vi "mock.vi"() -> ()   [LabVIEW 2017]
uses:
  refnum_array_cluster.ctl
  Utility Sub VIs/pulse_generator_data_charts.ctl
  Utility Sub VIs/pulse_generator_data.ctl
  Utility Sub VIs/pressure_temp_mixture.ctl
  Utility Sub VIs/diode_charts.ctl
panel:
  out "Diode Charts":T1
  out "Pressure/Temperature/Mixture Properties":T2
  out "Measurements":T3={"PG Abs Pressure"=119484.80284900061, "Vapor Temperature"=19.805676371442082, "Liquid Temperature"=19.52526901660894, "Tinlet"=121.24568157832624, "Tsectwo"=119.96937909943745, "TS Abs Pressure W1"=121.24568157832624, "TS Abs Pressure W7"=119.96937909943745, "W1-4 dP[Pa]"=19.52526901660894, "W1-7 dP[Pa]"=119.96937909943745, "W1-7 dP[Pa] Fast"=119.96937909943745, "PG Venturi dP [Pa]"=119.96937909943745, "Vapor Line Pitot dP [Pa]"=119.96937909943745, "Tsecthree"=19.191961040039615, "Toutlet"=19.148186089917207, "TS Ext"=18.97439824494449, "Vapor Sat Pressure"=121.24568157832624, "Liquid Sat Pressure"=119.96937909943745, "PG Mass Flow Rate"=nan, "Vapor Line Mass Flow"=119.96937909943745}
  out "Pulse Generator Charts":T4
  # "Saturation\nPressure [Pa]"
  # "Saturation\nTemperature [C]"
  # "Pressure [Pa]"
  # "Temperature [C]"
  # "Liquid Tank"
  # "Separator"
  # "Liquid Inlet"
  # "Vapor Tank"
  # "Vapor Inlet"
  # "Test Section"
  # "Upper Dev Section"
  # "Lower Dev Section"
  # "Test Section"
  # "Pulse Gen"
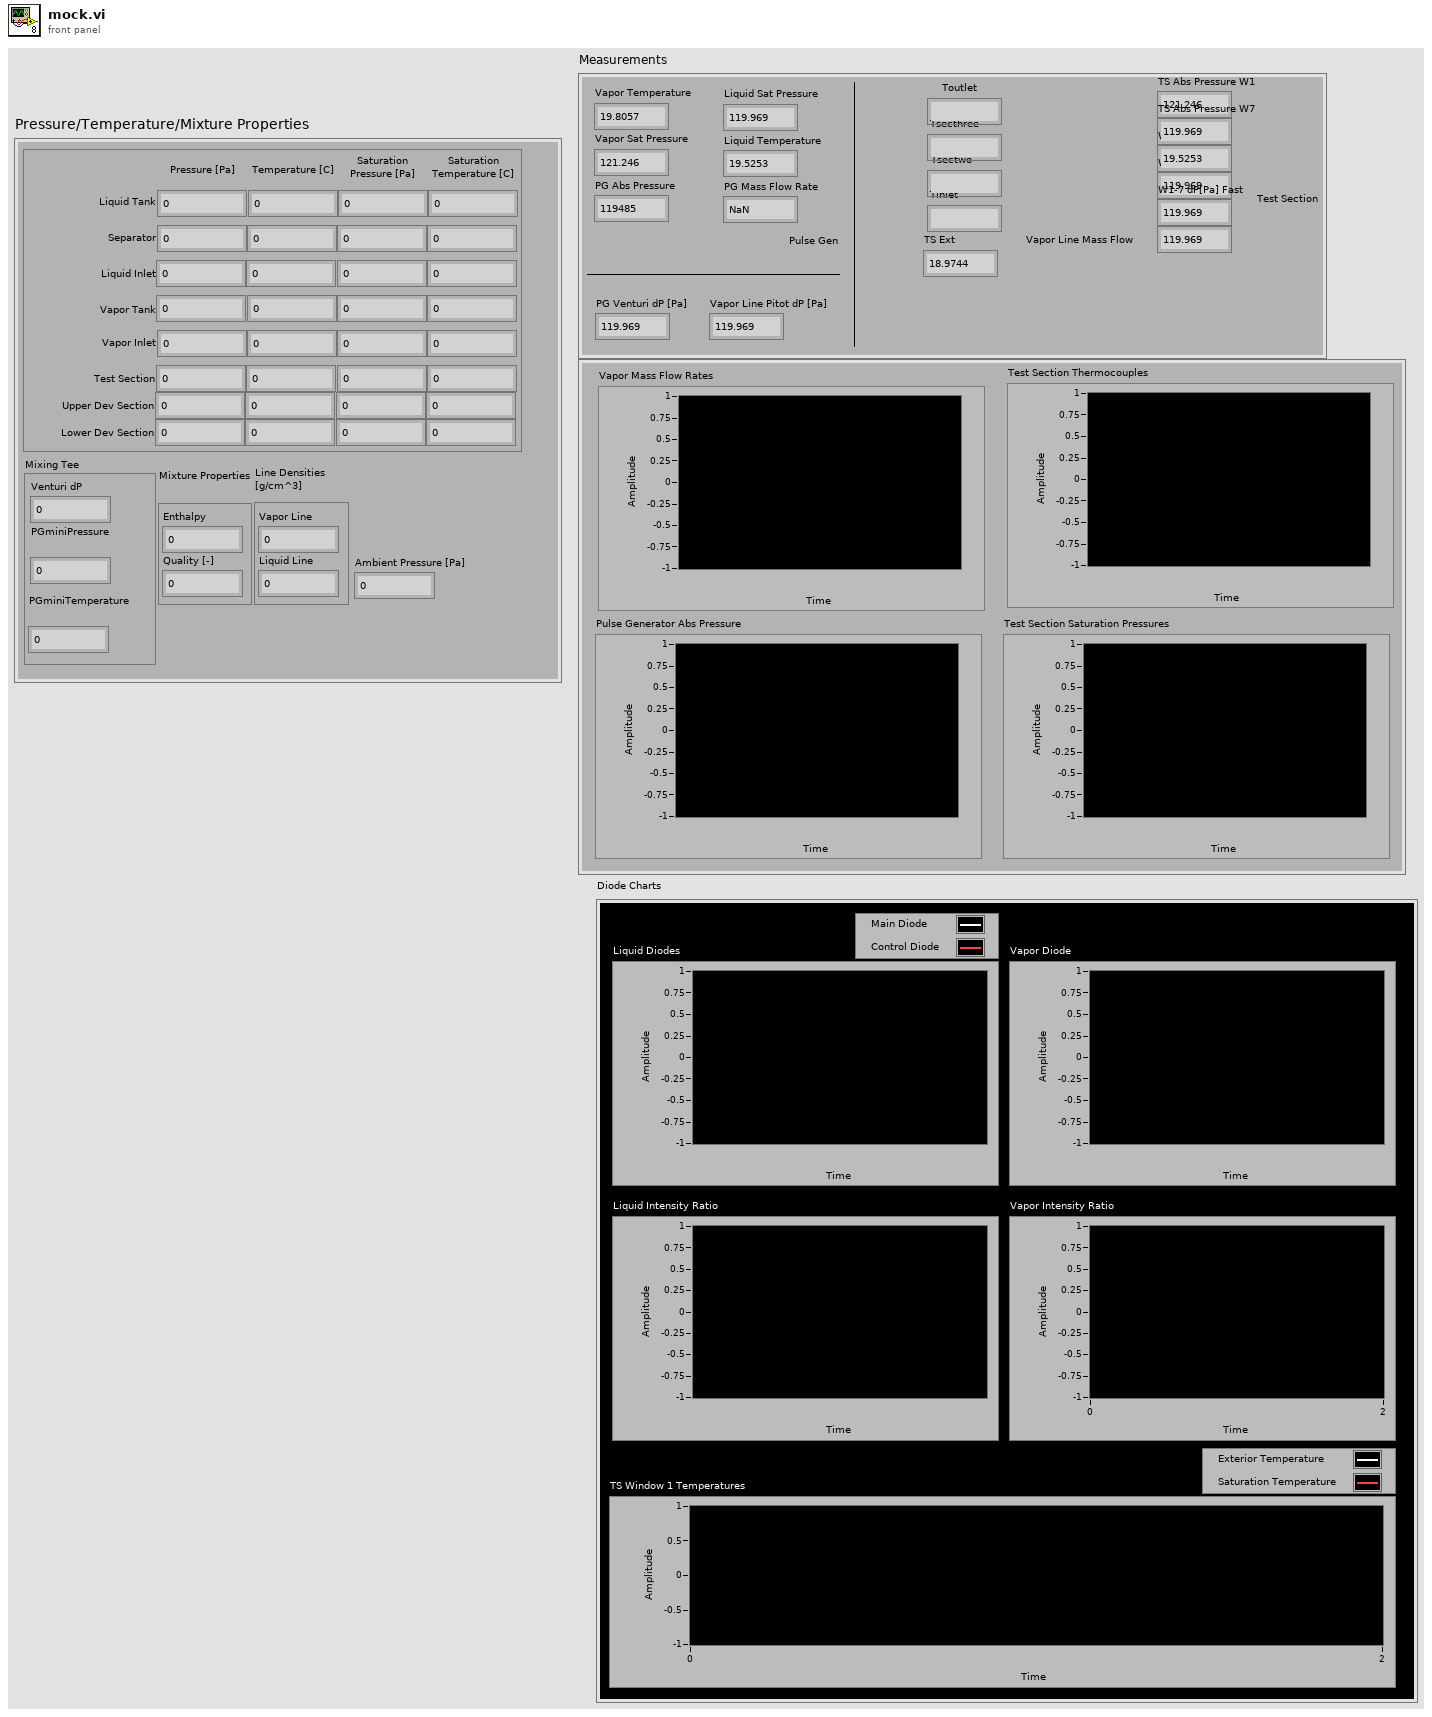
[diagram p1: front panel]
types:
  T1 = typedef "diode_charts.ctl" = cluster{"Liquid Diodes":cluster{dbl, dbl}, "Liquid Intensity Ratio":dbl, "Vapor Diode":cluster{dbl, dbl}, "Vapor Intensity Ratio":dbl, "TS Window 1 Temperatures":cluster{"Average":dbl, "T Sat [C]":dbl}}
  T2 = typedef "pressure_temp_mixture.ctl" = cluster{"Line Densities\n[g/cm^3]":cluster{"Vapor Line":dbl, "Liquid Line":dbl}, "Mixture Properties":cluster{"Enthalpy":dbl, "Quality [-]":dbl}, "Component PTs":cluster{"Liquid Tank P":dbl, "Liquid Tank T":dbl, "Liquid Tank Sat P":dbl, "Liquid Tank Sat T":dbl, "Separator P":dbl, "Separator T":dbl, "Separator Sat P":dbl, "Separator Sat T":dbl, "Liquid Inlet P":dbl, "Liquid Inlet T":dbl, "Liquid Inlet Sat P":dbl, "Liquid Inlet Sat T":dbl, "Vapor Tank P":dbl, "Vapor Tank T":dbl, "Vapor Tank Sat P":dbl, "Vapor Tank Sat T":dbl, "Vapor Inlet P":dbl, "Vapor Inlet T":dbl, "Vapor Inlet Sat P":dbl, "Vapor Inlet Sat T":dbl, "Test Section P":dbl, "Test Section T":dbl, "Test Section Sat P":dbl, "Test Section Sat T":dbl, "Upper Dev Section P":dbl, "Upper Dev Section T":dbl, "Upper Dev Section Sat P":dbl, "Upper Dev Section Sat T":dbl, "Lower Dev Section P":dbl, "Lower Dev Section T":dbl, "Lower Dev Section Sat P":dbl, "Lower Dev Section Sat T":dbl}, "Ambient Pressure [Pa]":dbl, "Mixing Tee":cluster{"Venturi dP":dbl, "PGminiPressure":dbl, "PGminiTemperature":dbl}}
  T3 = typedef "pulse_generator_data.ctl" = cluster{"PG Abs Pressure":dbl, "Vapor Temperature":dbl, "Liquid Temperature":dbl, "Tinlet":dbl, "Tsectwo":dbl, "TS Abs Pressure W1":dbl, "TS Abs Pressure W7":dbl, "W1-4 dP[Pa]":dbl, "W1-7 dP[Pa]":dbl, "W1-7 dP[Pa] Fast":dbl, "PG Venturi dP [Pa]":dbl, "Vapor Line Pitot dP [Pa]":dbl, "Tsecthree":dbl, "Toutlet":dbl, "TS Ext":dbl, "Vapor Sat Pressure":dbl, "Liquid Sat Pressure":dbl, "PG Mass Flow Rate":dbl, "Vapor Line Mass Flow":dbl}
  T4 = typedef "pulse_generator_data_charts.ctl" = cluster{"Vapor Mass Flow Rates":cluster{"max value":dbl, "max value":dbl}, "Test Section Thermocouples":cluster{"[0]":dbl, "[1]":dbl, "[2]":dbl, "[3]":dbl, "[4]":dbl}, "Pulse Generator Abs Pressure":dbl[], "Test Section Saturation Pressures":cluster{"max value":dbl, "max value":dbl}}
  T5 = typedef "refnum_array_cluster.ctl" = cluster{"Refnum Array":refnum<vi>[]}
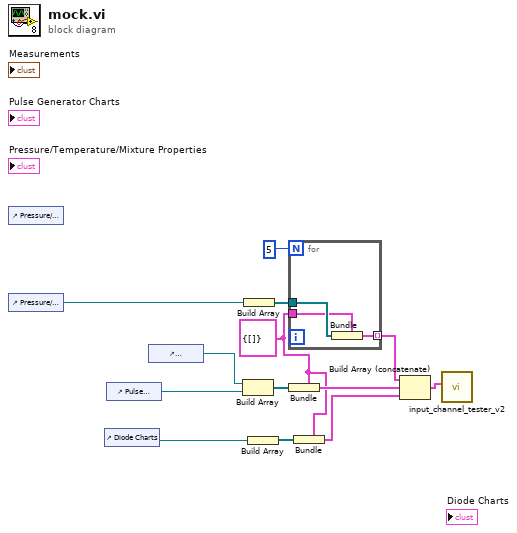
[diagram p0: block diagram]
diagram:
  w4 = T5 {"Refnum Array"=[]} ("Refnum Array Cluster")
  n1 = control-ref of="Pressure/Temperature/Mixture Properties"() -> ()  [unwired: 1 out]
  n2 = control-ref of="Pressure/Temperature/Mixture Properties"() -> (w8:refnum<vi>)
  n3 = control-ref of="Diode Charts"() -> (w3:refnum<vi>)
  n4 = control-ref of="Pulse Generator Charts"() -> (w12:refnum<vi>)
  n5 = control-ref of="Measurements"() -> (w13:refnum<vi>)
  n6 = Build Array(w13, w12) -> (w11:refnum<vi>[])
  n7 = Build Array(w8) -> (w6:refnum<vi>[])
  n8 = Build Array(w3) -> (w2:refnum<vi>[])
  n9 = for {
    N: 5 -> [_]
    tunnel: w6 -> [w15]
    tunnel: [w16] -> w5 mode=indexing
    tunnel: w4 -> [w14]
    n10 = Bundle(cluster=w14, "Refnum Array"=w15) -> (w16:T5)
  }
  n11 = Bundle(cluster=w4, "Refnum Array"=w11) -> (w10:T5)
  n12 = Bundle(cluster=w4, "Refnum Array"=w2) -> (w1:T5)
  n13 = Build Array (concatenate)(w5, w10, w1) -> (w9:T5[])
  n14 = call "input_channel_tester_v2.vi"("Refnums of Controls"=w9) -> ()  [unwired: 11 in]
